vi "Start FPGA DMA.vi"(8 "error in (no error)":errorcluster, 11 "FPGA VI Reference":T1) -> (0 "error out":errorcluster, 1 "Wait on IRQ Timeout?":bool, 3 "FPGA VI Reference":T1)   [LabVIEW 2014]
uses:
  controls/FPGA VI Reference.ctl
  <vilib>/Utility/error.llb/Error Cluster From Error Code.vi
  <vilib>/RVI Host/nirviSupport.llb/nirviErrorClusterFromErrorCode.vi
  <vilib>/rvi/errors/niLvFpgaAdjustHostInterfaceError.vi
  <vilib>/rvi/interface/nirviMethod/nirviMethod.xnode
  <vilib>/rvi/interface/nirviMethod/StockFPGA_InlinedMethodWaitForSingleIRQ.vi
  <vilib>/FPGAPlugInAG/Dynamic/niLvFpga_WaitOnIrq_Dynamic.vi
  <vilib>/FPGAPlugInAG/Dynamic/niLvFpga_AcknowledgeIrq_Dynamic.vi
  <vilib>/FPGAPlugInAG/Dynamic/niLvFpga_StartFifo_Dynamic.vi
  <vilib>/rvi/errors/niLvFpgaMergeErrorWithErrorCode.vi
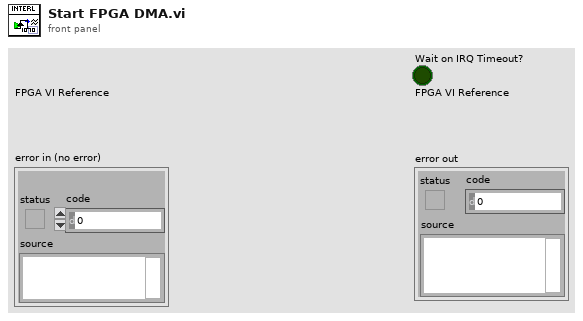
[diagram p1: front panel]
types:
  T1 = typedef "FPGA VI Reference.ctl" = refnum<k20>
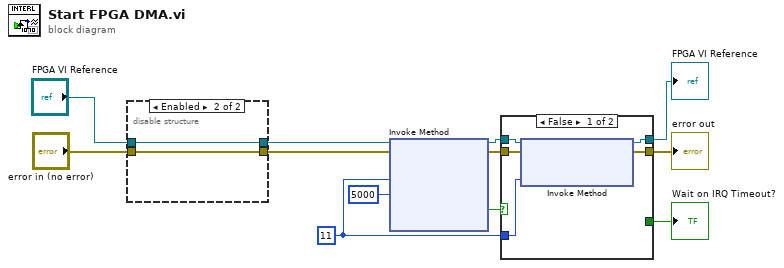
[diagram p0: block diagram]
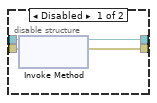
[diagram p2: hidden frame]
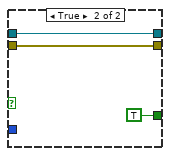
[diagram p3: hidden frame]
diagram:
  w4 = 11
  n1 = disable-structure shown="Enabled" {
    disable-tunnel: [w16 w17] -> w6
    disable-tunnel: [w15 w18] -> w5
    disable-tunnel: "error in (no error)" -> [w14 w17]
    disable-tunnel: "FPGA VI Reference" -> [w13 w18]
    frame Disabled {
      n2 = xnode "Invoke Method"("FPGA VI Reference In"=w13, "error in"=w14) -> ("FPGA VI Reference Out"=w15:T1, "error out"=w16:errorcluster)
    }
    frame Enabled {
    }
  }
  n3 = xnode "Invoke Method"("FPGA VI Reference In"=w5, "error in"=w6, "IRQ Number(s)"=w4, "Timeout (ms)"=5000) -> ("FPGA VI Reference Out"=w7:T1, "error out"=w8:errorcluster, "Timed Out"=w10:bool)  [unwired: 1 out]
  n4 = case shown="False" w10 {
    tunnel: w7 -> [w23 w24]
    tunnel: w8 -> [w22 w26]
    tunnel: [w21 w26] -> w11
    tunnel: w4 -> [w20 _]
    tunnel: [_ TRUE] -> w12
    tunnel: [w19 w24] -> w2
    frame False {
      n5 = xnode "Invoke Method"("FPGA VI Reference In"=w23, "error in"=w22, "IRQ Number(s)"=w20) -> ("FPGA VI Reference Out"=w19:T1, "error out"=w21:errorcluster)
    }
    frame True {
    }
  }
  "Wait on IRQ Timeout?" <- w12
  "error out" <- w11
  "FPGA VI Reference" <- w2
